vi "AddFilter.vi"(8 "Error in (no error)":errorcluster, 10 "LogFilterInterface in":refnum<class "LogFilterInterface.lvclass">, 11 "LogWriterInterface in":refnum<class "LogWriterInterface.lvclass">) -> (0 "Error out":errorcluster, 3 "LogWriterInterface out":refnum<class "LogWriterInterface.lvclass">)   [LabVIEW 2011, in "LogWriterInterface.lvclass"]
uses:
  LogWriterInterface.lvclass
  Filter/LogFilterInterface/LogFilterInterface.lvclass
  LogWriterInterface.lvclass/LogWriterInterface.ctl
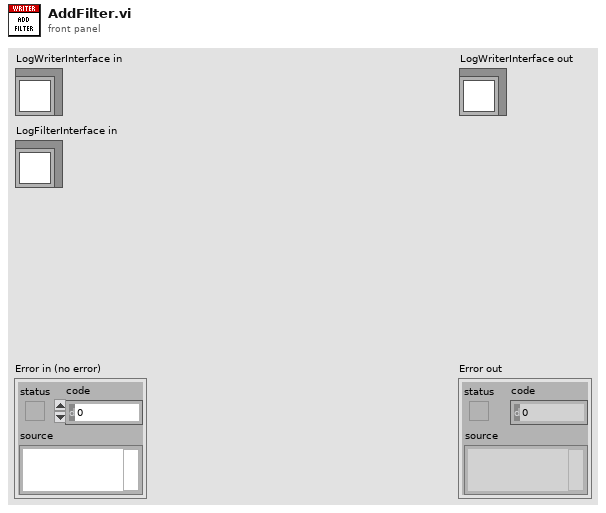
[diagram p1: front panel]
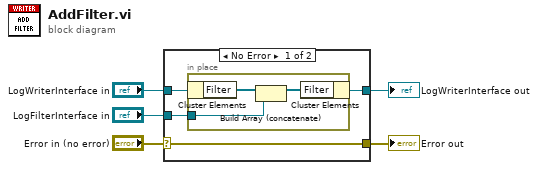
[diagram p0: block diagram]
diagram:
  n1 = case shown="No Error" "Error in (no error)" {
    selector: "Error in (no error)" -> [w9 w13]
    tunnel: [w9 w13] -> w4
    tunnel: [w6 w14] -> w2
    tunnel: "LogWriterInterface in" -> [w8 w14]
    tunnel: "LogFilterInterface in" -> [w7 _]
    frame No Error {
      n2 = in-place {
        in-place-border: w7 -> [w10]
        n3 = in-place-cluster #1(w8) -> ("Filter"=w12:refnum<class "LogFilterInterface.lvclass">[])
        n4 = Build Array (concatenate)(w12, w10) -> (w11:refnum<class "LogFilterInterface.lvclass">[])
        n5 = in-place-cluster #1("Filter"=w11) -> (w6:refnum<class "LogWriterInterface.lvclass">)
      }
    }
    frame Error {
    }
  }
  "Error out" <- w4
  "LogWriterInterface out" <- w2
